vi "ReadRoomsNumbers.vi"(8 "error in (no error)":errorcluster) -> (0 "error out":errorcluster, 2 "RoomNumbers":i32[](array[numeric]))   [LabVIEW 2015, in "RestApi.lvlib"]
uses:
  RestApi.lvlib
  TypeDef/GetRoomCommands.ctl
panel:
  out "JSON":string
  # "http://127.0.0.1:8001/WebService1/ReadFlag?Room={value}"
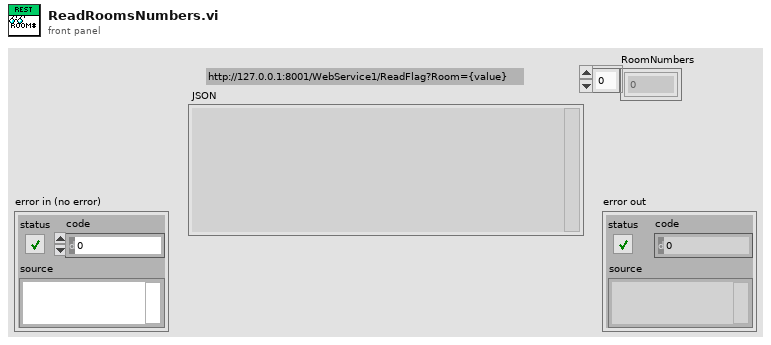
[diagram p1: front panel]
types:
  T1 = typedef "RestApi.lvlib/GetRoomCommands.ctl" = enum16{"ReadRoom", "ReadFlag", "ReadFlagState", "ReadFlagColor", "ReadBedVacant", "ReadPersonnel", "ReadRequests", "ReadBeaconID", "ReadBedURL", "ReadRoomsNumbers"}
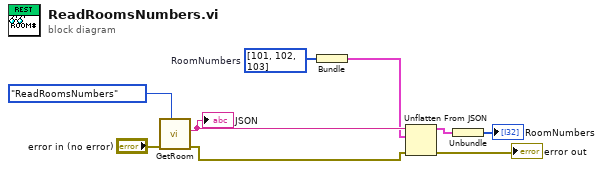
[diagram p0: block diagram]
diagram:
  w7 = i32[] [101, 102, 103]  # RoomNumbers
  n1 = call "GetRoom.vi"("Room Commands"=GetRoomCommands."ReadRoomsNumbers", "error in (no error)"="error in (no error)") -> ("error out"=w4:errorcluster, "Flags JSON"=w6:string)  [unwired: 8 in]
  "JSON" <- w6
  n2 = Bundle("RoomNumbers"=w7) -> (w5:cluster{"RoomNumbers":i32[]})  [unwired: 1 in]
  n3 = Unflatten From JSON(JSON string=w6, type and defaults=w5, error in (no error)=w4) -> (value=w2:cluster{"RoomNumbers":i32[]}, error out=→"error out":errorcluster)  [unwired: 4 in]
  n4 = Unbundle(w2) -> ("RoomNumbers"=→"RoomNumbers":i32[])
